vi "Tree to Structure.vi"(8 "error in":errorcluster, 10 "Structure Branch In":refnum<class "Tree.lvclass">, 11 "Tree In":refnum<class "Tree.lvclass">) -> (0 "error out":errorcluster, 2 "Structure Branch Out":refnum<class "Tree.lvclass">, 3 "Tree out":refnum<class "Tree.lvclass">)   [LabVIEW 2019]
uses:
  Tree/Tree.lvclass
  TypeDefs/STRUCTURE.ctl
  TypeDefs/ELEMENT.ctl
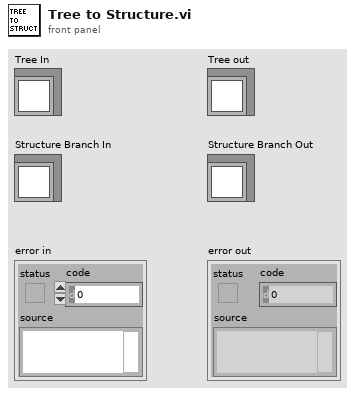
[diagram p1: front panel]
types:
  T1 = typedef "ELEMENT.ctl" = cluster{"DATATYPE":i16, "LAYER":i16, "XY":cluster{"X":i32[], "Y":i32[]}, "SREF":cluster{"Is SREF":bool, "REF":string}}
  T2 = typedef "STRUCTURE.ctl" = cluster{"ELEMENTS":T1[], "NAME":string}
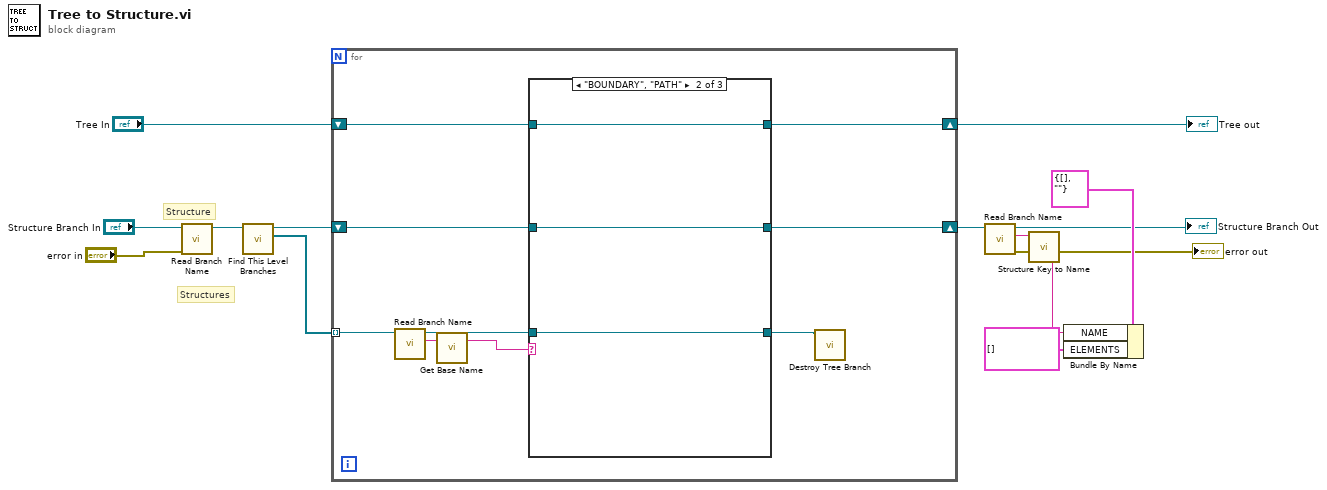
[diagram p0: block diagram]
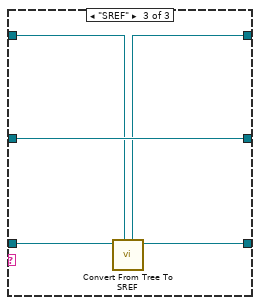
[diagram p3: hidden frame]
diagram:
  # "Structure"
  # "Structures"
  n1 = call "Read Branch Name.vi"("error in"="error in", "Tree in"="Structure Branch In") -> ("Tree out"=w14:refnum<class "Tree.lvclass">)  [unwired: 7 in, 2 out]
  n2 = call "Find This Level Branches.vi"("Tree in"=w14) -> ("Branches"=w7:refnum<class "Tree.lvclass">[], "Tree out"=w12:refnum<class "Tree.lvclass">)  [unwired: 8 in, 1 out]
  n3 = for {
    shift-right: [w20] -> w13
    shift-left: "Tree In" -> [w21]
    tunnel: w7 -> [w23] mode=indexing
    shift-right: [w18] -> w11
    shift-left: w12 -> [w19]
    n4 = call "Read Branch Name.vi"("Tree in"=w23) -> ("Branch Name"=w22:string, "Tree out"=w16:refnum<class "Tree.lvclass">)  [unwired: 8 in, 1 out]
    n5 = call "Get Base Name.vi"("Unique Name"=w22) -> ("Base Name"=w17:string)  [unwired: 2 in]
    n6 = case shown="\"BOUNDARY\", \"PATH\"" w17 {
      tunnel: w21 -> [w26 w29 w30]
      tunnel: [w26 w29 w31] -> w20
      tunnel: w19 -> [w25 w28 w34]
      tunnel: [w25 w28 w34] -> w18
      tunnel: w16 -> [w24 w27 w32]
      tunnel: [w24 w27 w33] -> w15
      frame Default {
      }
      frame "BOUNDARY", "PATH" {
      }
      frame "SREF" {
        n7 = call "Convert From Tree To SREF.vi"("Root In"=w30, "Branch in"=w32) -> ("Branch out"=w33:refnum<class "Tree.lvclass">, "Root Out"=w31:refnum<class "Tree.lvclass">)  [unwired: 7 in, 1 out]
      }
    }
    n8 = call "Destroy Tree Branch.vi"("Tree in"=w15) -> ()  [unwired: 9 in, 2 out]
  }
  "Tree out" <- w13
  n9 = call "Read Branch Name.vi"("Tree in"=w11) -> ("error out"=→"error out":errorcluster, "Branch Name"=w9:string, "Tree out"=→"Structure Branch Out":refnum<class "Tree.lvclass">)  [unwired: 8 in]
  n10 = call "Structure Key to Name.vi"("Key"=w9) -> ("Name"=w8:string)  [unwired: 4 in]
  n11 = Bundle By Name(cluster=T2 {"ELEMENTS"=[], "NAME"=""} ("STRUCTURE"), "NAME"=w8, "ELEMENTS"=T1[] []) -> ()  [unwired: 1 out]
